vi "WholeImageROIFit.vi"(3 "Select directory with EYE files":path=path "E:/Focus Surgery/TTI LV Core") -> ()   [LabVIEW 2022 SP3]
uses:
  ViewData/-ReadEye/ScaleMethod.ctl
  <vilib>/Analysis/baseanly.llb/Mean (DBL).vi
  <vilib>/Utility/file.llb/Read Delimited Spreadsheet (DBL).vi
  <vilib>/Utility/file.llb/Write Delimited Spreadsheet (DBL).vi
  <vilib>/Analysis/NI_AALBase.lvlib
panel:
  out "Waveform Graph":cluster{"x-y":dbl, dbl, dbl[][]}(graph)
  out "spe vs depth":dbl[][](array[numeric])
  out "FileName":string
  in  "Color Scale":u16(ring) items=["Grey Scale", "Color Scale"]
  out "Sector as data array":dbl[][](graph)
  out "min value":dbl
  out "max value":dbl
  in  "ExitSendCmd":bool
  in  "Calculate TTIs":bool
  out "Current File":string
  out "Col scores":dbl[][](graph)
  out "Col midband":dbl[][](graph)
  out "NN Score":dbl[][](graph)
  in  "Tab Control":T1(tab)=enum."NNScore"
  in  "Type of Mean":u16(ring) items=["Mean from lines", "Mean just lines", "Poly Mean", "No mean", "Filter"]
  in  "Corrections":T2(ring)=enum."att correction"
  in  "type of cal file":u16(ring) items=["Normal Cal File", "Cross Cal File", "No cal file"]
  out "Cal File Att":string
  out "RF File Att":string
  out "Cal File Name":string
  in  "Fit band":T3 {"center freq" format="%.2f"; "stop freq" format="%.2f"; "start" format="%.2f"}
  in  "Use Info In Header?":bool=TRUE
  in  "Lines to Avg":i32=1
  in  "Pts between window":i32=8
  in  "Pts in window":i32=64
  in  "sound speed":dbl=1.5 format="%.2f"
  in  "Padded FFT size":u16(ring)=6 items=["next 2^n", "8", "16", "32", "64", "128", "256", "512"]
  in  "Att (db/ cm MHz)":dbl=0.5 format="%.2f"
  in  "Add Switch Noise?":bool
  in  "Log scaling?":T4=enum."Log Grey Scale"
  out "Fit array":T5
  in  "Define Att Start":bool
  out "window in mm":dbl
  in  "Axis scaling":bool
  out "dist between windows in mm":dbl
  in  "Sub-Band Filter":T6={"Fit band"={"low freq"=3.5, "high freq"=8.0, "center freq"=5.75}, "MB threshold"=0.0, "Sub-Band Filter?"=FALSE} {"MB threshold" format="%.2f"; "Fit band"."center freq" format="%.2f"; "Fit band"."high freq" format="%.2f"; "Fit band"."low freq" format="%.2f"}
  in  "Filter Prams":T7={"low cutoff"=5, "order"=81, "high cutoff"=35}
  in  "CQPrams":T8={"Data System params"={"sample freq (MHz)"=50.0, "focal length (mm)"=32.0, "aperature radius (mm)"=3.5, "pts in window"=64.0}, "Show CQ^2 image?"=FALSE, "Save?"=FALSE} {"Data System params"."pts in window" format="%.2f"; "Data System params"."aperature radius (mm)" format="%.2f"; "Data System params"."focal length (mm)" format="%.2f"; "Data System params"."sample freq (MHz)" format="%.2f"}
  out "CQ^2":ext[][](graph)
  out "radius (micron)":sgl[][](graph)
  in  "Range Params":T9={"mb max"=-20.0, "mb min"=-70.0, "slope max"=8.0, "slope min"=-8.0, "int max"=5.0, "int min"=-85.0} {"int min" format="%.2f"; "int max" format="%.2f"; "slope min" format="%.2f"; "slope max" format="%.2f"; "mb min" format="%.2f"; "mb max" format="%.2f"}
  in  "Final Sector Image Size":T10={"x"=346, "y"=240, "Trim image sides?"=FALSE, "start trim"=45, "end trim line"=256}
  in  "Simple BMP":bool
  in  "Raw Data Formats":T11(ring)
  in  "Save Raw Results?":bool
  out "inc x (mm)":dbl format="%.3f"
  out "inc y (mm)":dbl format="%.3f"
  out "Range Params in LUT":T9 {"int min" format="%.2f"; "int max" format="%.2f"; "slope min" format="%.2f"; "slope max" format="%.2f"; "mb min" format="%.2f"; "mb max" format="%.2f"}
  in  "Bypass Sector?":bool
  in  "PSA Value":dbl=8.7 format="%.2f"
  in  "Look Up Table":path=path "E:/Focus Surgery/TTI LV Core/99lktbl10-31.dat"
  in  "Create Score Image?":bool
  in  "thresholds":T12={"T1"=0.37, "T2"=0.38, "T3"=0.39, "T4"=0.4, "T5"=0.43} {"T5" scale=-0.1442227..0.5211197 scale format="%#_1g"; "T4" scale=-0.1442227..0.5211197 scale format="%#_1g"; "T3" scale=-0.1442227..0.5211197 scale format="%#_1g"; "T2" scale=-0.1442227..0.5211197 scale format="%#_1g"; "T1" scale=-0.1442227..0.6 scale format="%#_1g"}
  in  "Save Score Dat?":bool
  in  "Color Table":u32[](array[colorbox])=[0, 0, 65793, 131586, 197379, 263172, 328965, 394758, 460551, 526344, 592137, 657930, 723723, 789516, 855309, 921102, 986895, 1052688, 1118481, 1184274, 1250067, 1315860, 1381653, 1447446, 1513239, 1579032, 1644825, 1710618, 1776411, 1842204, 1907997, 1973790, 2039583, 2105376, 2171169, 2236962, 2302755, 2368548, 2434341, 2500134, 2565927, 2631720, 2697513, 2763306, 2829099, 2894892, 2960685, 3026478, 3092271, 3158064, 3223857, 3289650, 3355443, 3421236, 3487029, 3552822, 3618615, 3684408, 3750201, 3815994, 3881787, 3947580, 4013373, 4079166, 4144959, 4210752, 4276545, 4342338, 4408131, 4473924, 4539717, 4605510, 4671303, 4737096, 4802889, 4868682, 4934475, 5000268, 5066061, 5131854, 5197647, 5263440, 5329233, 5395026, 5460819, 5526612, 5592405, 5658198, 5723991, 5789784, 5855577, 5921370, 5987163, 6052956, 6118749, 6184542, 6250335, 6316128, 6381921, 6447714, 6513507, 6579300, 6645093, 6710886, 6776679, 6842472, 6908265, 6974058, 7039851, 7105644, 7171437, 7237230, 7303023, 7368816, 7434609, 7500402, 7566195, 7631988, 7697781, 7763574, 7829367, 7895160, 7960953, 8026746, 8092539, 8158332, 8224125, 8289918, 8355711, 8421504, 8487297, 8553090, 8618883, 8684676, 8750469, 8816262, 8882055, 8947848, 9013641, 9079434, 9145227, 9211020, 9276813, 9342606, 9408399, 9474192, 9539985, 9605778, 9671571, 9737364, 9803157, 9868950, 9934743, 10000536, 10066329, 10132122, 10197915, 10263708, 10329501, 10395294, 10461087, 10526880, 10592673, 10658466, 10724259, 10790052, 10855845, 10921638, 10987431, 11053224, 11119017, 11184810, 11250603, 11316396, 11382189, 11447982, 11513775, 11579568, 11645361, 11711154, 11776947, 11842740, 11908533, 11974326, 12040119, 12105912, 12171705, 12237498, 12303291, 12369084, 12434877, 12500670, 12566463, 12632256, 12698049, 12763842, 12829635, 12895428, 12961221, 13027014, 13092807, 13158600, 13224393, 13290186, 13355979, 13421772, 13487565, 13553358, 13619151, 13684944, 13750737, 13816530, 13882323, 13948116, 14013909, 14079702, 14145495, 14211288, 14277081, 14342874, 14408667, 14474460, 14540253, 14606046, 14671839, 14737632, 14803425, 14869218, 14935011, 15000804, 15066597, 15132390, 15198183, 15263976, 15329769, 15395562, 15461355, 15527148, 15592941, 15658734, 15724527, 15790320, 15856113, 15921906, 15987699, 16053492, 16119285, 16185078, 16250871, 16316664, 16382457, 6352640, 12058434, 16770066, 16758546, 16711731]
  in  "Data Set":i32
  in  "Rescale Thresh":bool
  in  "Save Cross Cal?":bool
  in  "Create Cross Cal?":bool
  out "Cross Cal":dbl[][](graph)
  in  "Avg #":i32=10
  out "avg":dbl[](array[numeric])
  in  "start avg":i32=270
  in  "AVG pts":i32=20
  in  "Save STFT AVG":bool
  in  "Ring":u16(ring) items=["Select Files in Listbox", "Choose list of files"]
  in  "File Names":i32[](listbox)
  out "raw data":i16[][](graph)
  out "midband fit":dbl[][](graph)
  out "intercept":dbl[][](graph)
  out "slope":dbl[][](graph)
  # "Z:\\_BIOMED_ARCHIVE\\Ex_Staff\\Andy_Kalisz_PC\\HITACHI\\HITACHI_2003-VMMC-CCal\\Andy_VMMC_2003-08-22_disk2\\Gel-cal\\EUP-V53W_End-Fire_Probe_SE13133935\\F3\\EYEfiles_-4dB"
  # "Z:\\_BIOMED_ARCHIVE\\DATA\\PROSTATE\\CALIBRATION AND X-CALIB\\NEW Data\\CrossCal Data - RRI Hitachi\\DG_2011-01-13"
  # "© 2000-2010 Riverside Research Institute"
  # "Parameters to select before hitting \"Calculate TTIs\"."
  # "Select to add back in switch noise from B&K Hawk machine."
  # "Spectrum Fit Parameters"
  # "Values used to make image."
  # "Optional suband filter which is really never used and may not function properly in current version."
  # "Can be selected after calculating TTIs"
  # "CQPrams files are saved as spreadsheet files. Radius file is in microns and cq^2 file is in dB."
  # "Pixel spacing of sector image.\n(Need to be same for 1:1 aspect ration.)"
  # "Save raw data and MB side by side"
  # "Score images need to be created with all corrections applied data. This means a cross cal file with attenutation corrections for Hawk and Hitachi, and data base corrections for B&K 3535.\n\nFinal image size settings are in Image Prams tab. Data saves as a BMP file in sector format.\n\nCreate Score Image? will color code images and Save Score Dat? will save images as BMPs."
  # "If making Cross Cal file, select No cal file option and att correction."
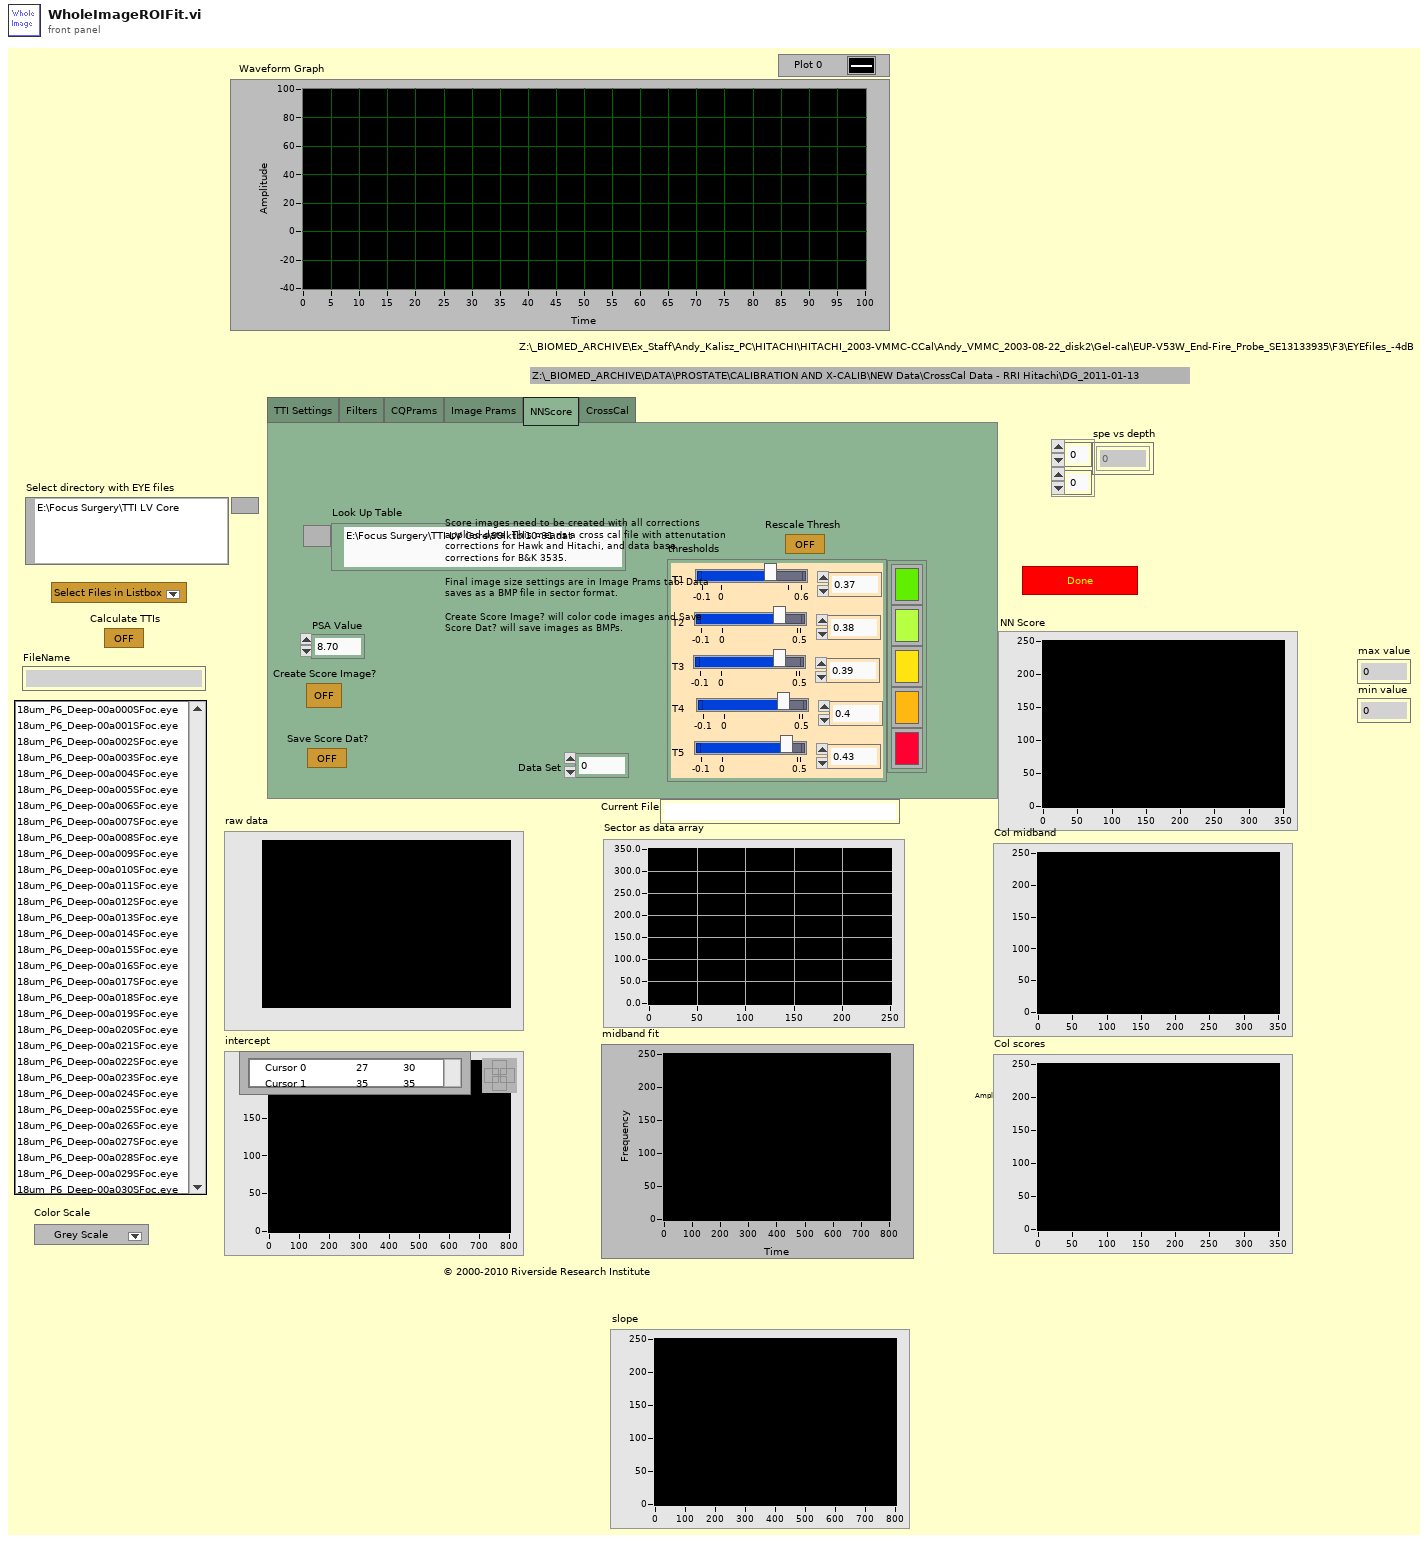
[diagram p1: front panel]
types:
  T1 = enum32{"TTI Settings", "Filters", "CQPrams", "Image Prams", "NNScore", "CrossCal"}
  T2 = enum16{"no att correction", "att correction", "B&K 3535, TGC & att corr"}
  T3 = cluster{"start":dbl, "stop freq":dbl, "center freq":dbl}
  T4 = typedef "ScaleMethod.ctl" = enum16{"Linear Abs Grey", "Log Grey Scale", "Linear Color Scale", "dB Scale", "Verasonics Doppler"}
  T5 = cluster{"x length":i32, "y length":i32, "ROIs in x":i32, "ROIs in y":i32}
  T6 = cluster{"Fit band":cluster{"low freq":dbl, "high freq":dbl, "center freq":dbl}, "MB threshold":dbl, "Sub-Band Filter?":bool}
  T7 = cluster{"low cutoff":i32, "order":i32, "high cutoff":i32}
  T8 = cluster{"Data System params":cluster{"sample freq (MHz)":dbl, "focal length (mm)":sgl, "aperature radius (mm)":sgl, "pts in window":dbl}, "Show CQ^2 image?":bool, "Save?":bool}
  T9 = cluster{"mb max":dbl, "mb min":dbl, "slope max":dbl, "slope min":dbl, "int max":dbl, "int min":dbl}
  T10 = cluster{"x":i32, "y":i32, "Trim image sides?":bool, "start trim":i32, "end trim line":i32}
  T11 = enum16{"spreadsheet", "8 bit byte file", "sector byte file", "8 bit BMP file", "sector 8 bit BMP file"}
  T12 = cluster{"T1":dbl, "T2":dbl, "T3":dbl, "T4":dbl, "T5":dbl}
  T13 = typedef "Header.ctl" = cluster{"header info":cluster{"Header":string, "Head length":i16}, "A/D info":cluster{"# rf points per line":u16, "# lines per scan":u16, "sample rate MHz":u16, "# A/D bits":i16, "# bytes per A/D":u16, "TGC Flag":u16, "A/D Type":string}, "Tranducer Info":cluster{"bandwidth":sgl, "center freq":sgl, "start freq":sgl, "ID":i32}, "Scan Info":cluster{"delay":sgl, "pivot distance":sgl, "sector scan angle":sgl, "operator":string, "Scan Mode":string, "location":string}, "Time/Date Info":cluster{"date":string, "time":string}, "RF Info":cluster{"RF file name":string, "RF file att":string, "RF cal file name":string, "RF cal file att":string}, "Patient Info":cluster{"ID":string, "extended ID":string, "age":u16, "sex":string, "previously\nscanned":string, "PSA":sgl, "LOS":u8, "Ethnicty 2":u8, "Race":u8}, "Tissue Type":cluster{"organ":i16, "disease type":i16, "disease location":i16, "IQ_pts":u16, "RcvBuffer":u8, "RcvFrame":u16, "IQBuff":u8, "IQFrame":u16, "IQPage":u8}, "Votage scaling":cluster{"Digitizer (dB)":sgl, "Gain (dB)":sgl, "Atten (dB)":sgl}, "Comment":string, "Misc Info":cluster{"avg num":u16, "c speed":i16, "Div By or SF zones":i16, "XMIT CHS":u8, "RCV CHS":u8, "Xmit angle":sgl}, "Therapy Parameters":cluster{"Theraputic Freq (MHz)":sgl, "Time on (s)":sgl, "Therapy amplitude (mV)":sgl, "Lines Before":u16, "Lines After":u16}, "Scan Settings":cluster{"Energy (uJ or V)":u8, "Damp (Ohm) or Fc":u8, "HP Filt (KHz)":u8, "LP Filt (MHz)":u8, "Gain (db)":u8, "prf (kHz)":sgl, "Distance between\nscan lines (um)":u16, "Distance between\nscan planes (um)":u16, "Scan line gap (um)":sgl, "Scan plane gap (um)":sgl}, "Compression Parameters":cluster{"F1 (MHz)":sgl, "F2 (MHz)":sgl, "% taper":sgl, "duration":sgl}, "Patient Info Xtra":cluster{"First Name":string, "Last Name":string, "Notes":string}, "ROI Box":u16[]}
  T14 = cluster{"delay":sgl, "pivot distance":sgl, "sector scan angle":sgl, "operator":string, "Scan Mode":string, "location":string}
  T15 = cluster{"X right":dbl, "X left":dbl, "Y low":dbl, "Y high":dbl}
  T16 = cluster{"RF file name":string, "RF File Att":string, "Cal File Name":string, "Cal File Att":string}
  T17 = cluster{"RF file name":string, "RF file att":string, "RF cal file name":string, "RF cal file att":string}
  T18 = cluster{"start freq":sgl, sgl, "center freq":sgl}
  T19 = cluster{"bandwidth":sgl, "center freq":sgl, "start freq":sgl, "ID":i32}
  T20 = cluster{"Pts in window":i32, "Lines to Avg":i32, dbl, "# lines per scan":u16}
  T21 = cluster{"slope (m)":dbl[][], "intercept (b)":dbl[][], "midband fit":dbl[][], "pts in fit":dbl}
  T22 = cluster{"slope (m)":dbl, "m stand dev":dbl, "intercept (b)":dbl, "b stand dev":dbl, "MSE":dbl, "midband fit":dbl, "pts in fit":dbl}
  T23 = typedef "imagedata.ctl" = cluster{"image type":i32, "image depth":i32, "image":u8[], "mask":u8[], "colors":u32[], "Rectangle":cluster{"left":i16, "top":i16, "right":i16, "bottom":i16}}
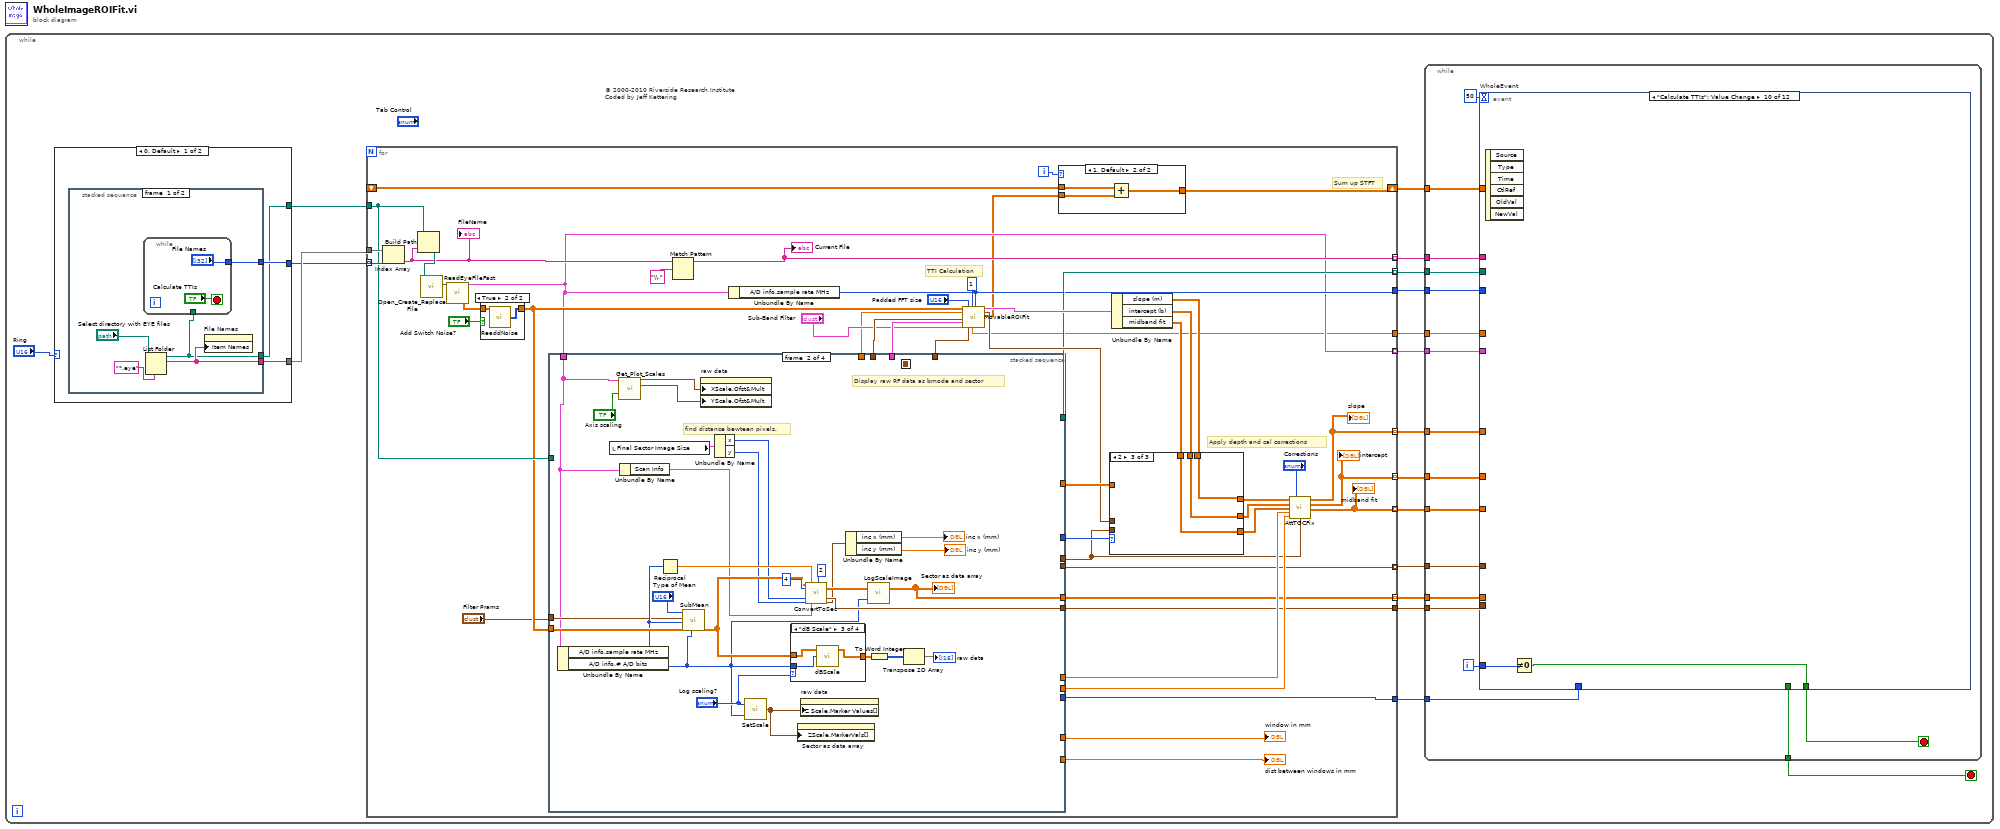
[diagram p0: block diagram]
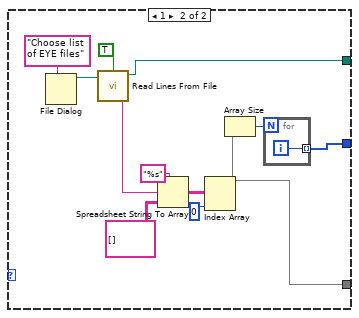
[diagram p3: hidden frame]
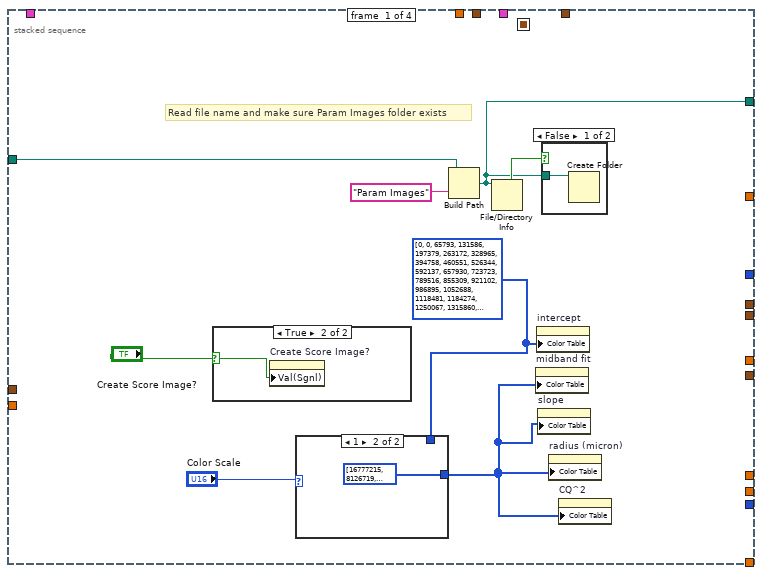
[diagram p5: hidden frame]
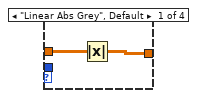
[diagram p9: hidden frame]
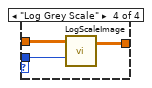
[diagram p11: hidden frame]
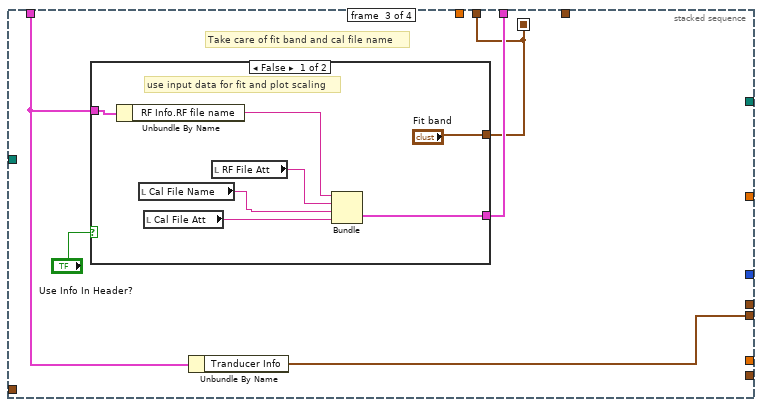
[diagram p12: hidden frame]
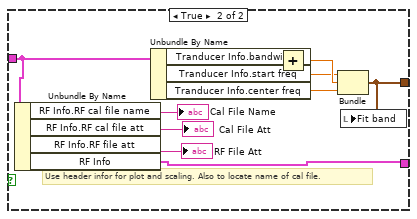
[diagram p13: hidden frame]
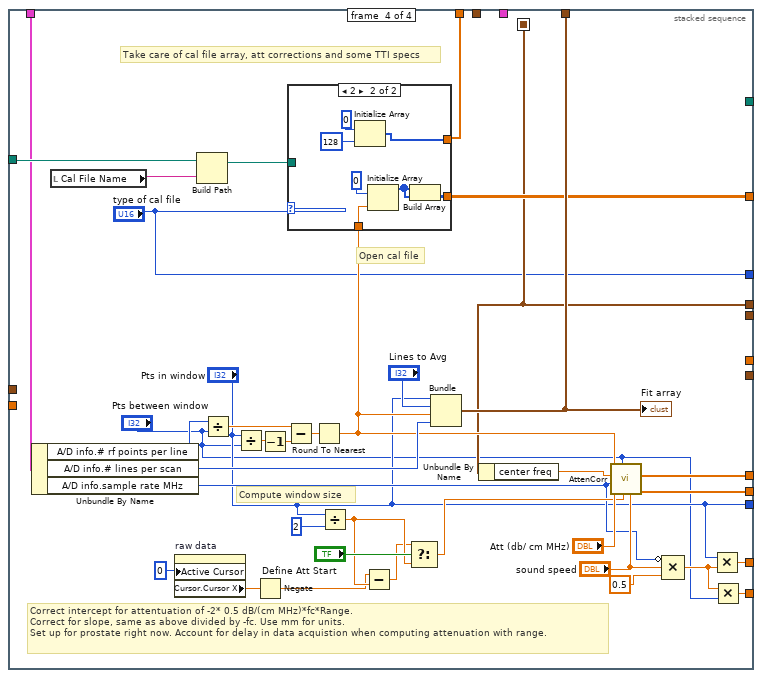
[diagram p14: hidden frame]
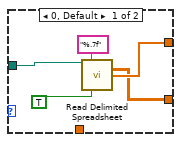
[diagram p15: hidden frame]
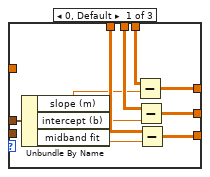
[diagram p17: hidden frame]
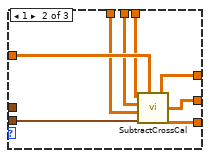
[diagram p18: hidden frame]
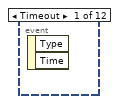
[diagram p19: hidden frame]
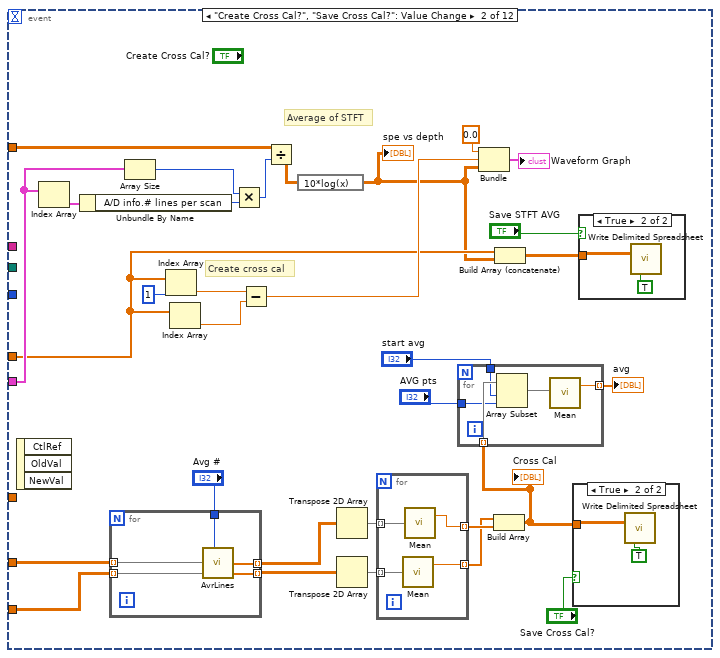
[diagram p20: hidden frame]
diagram:
  n1 = while {
    stop <- w5 stop-if-true
    # "© 2000-2010 Riverside Research Institute\nCoded by Jeff Kettering"
    n2 = case shown="0, Default" "Ring" {
      tunnel: [w21 w31] -> w18
      tunnel: [w20 w30] -> w17
      tunnel: [w19 w29] -> w4
      frame 0, Default {
        n3 = stacked-sequence {
          tunnel: [w23 _] -> w21
          tunnel: [w24 _] -> w20
          tunnel: [w22 _] -> w19
          frame #0 {
            n4 = List Folder(path="Select directory with EYE files", pattern="*.eye") -> (path out=w22:path, filenames=w23:string[])  [unwired: 1 in, 3 out]
            n5 = while {
              tunnel: ["File Names"] -> w24
              tunnel: w22 -> [_]
              stop <- "Calculate TTIs" stop-if-true
            }
            n6 = property on="File Names" class="LstBox (strict)"("Item Names"=w23) -> ()  [unwired: 2 in, 2 out]
          }
          frame #1 {
          }
        }
      }
      frame 1 {
        n7 = File Dialog(7:"Choose list of EYE files" ("prompt")) -> (3:w38:path)  [unwired: 1 in, 8 out]
        n8 = call <vilib>:"Read Lines From File.vi"("convert eol? (no:F)"=TRUE, "file path (dialog if empty)"=w38) -> ("new file path (Not A Path if cancelled)"=w29:path, "line string"=w33:string)  [unwired: 1 in, 5 out]
        n9 = Spreadsheet String To Array(format string="%s", spreadsheet string=w33, array type (2D Dbl)=string[][] [] ("Array Constant")) -> (array=w37:string[][])  [unwired: 1 in]
        n10 = Index Array(array=w37, index (col)=0) -> (element=w31:string[])  [unwired: 1 in]
        n11 = Array Size(array=w31) -> (size(s)=w32:i32)
        n12 = for {
          N: w32 -> [_]
          tunnel: [w41] -> w30 mode=indexing
          i -> [w41]
        }
      }
    }
    n13 = for {
      tunnel: w18 -> [w88]
      tunnel: w4 -> [w66]
      tunnel: w17 -> [w86] mode=indexing
      tunnel: [w60] -> w16 mode=indexing
      tunnel: [w67] -> w15 mode=indexing
      tunnel: [w56] -> w14 mode=indexing
      tunnel: [w54] -> w13 mode=indexing
      tunnel: [w68] -> w12 mode=indexing
      tunnel: [w55] -> w11 mode=indexing
      tunnel: [w51] -> w10 mode=indexing
      tunnel: [w65] -> w9
      tunnel: [w59] -> w8 mode=indexing
      tunnel: [w52] -> w7
      tunnel: [w57] -> w6
      shift-right: [w42] -> w2
      shift-left: _ -> [w47]
      tunnel: [w49] -> w1
      i -> [w46]
      # "Sum up STFT"
      # "Apply depth and cal corrections"
      # "TTI Calculation"
      n14 = Index Array(array=w88, index=w86) -> (element=w61:string)
      "FileName" <- w61
      n15 = Build Path(base path=w66, name or relative path=w61) -> (appended path=w87:path)
      n16 = call <vilib>:"Open_Create_Replace File.vi"("file path"=w87) -> ("new file path"=w72:path)  [unwired: 5 in, 5 out]
      n17 = call "ReadEyeFileFast.vi"("new file path"=w72) -> ("2-D data array"=w58:sgl[][], "Header In"=w51:T13)  [unwired: 13 in, 4 out]
      n18 = case shown="True" "Add Switch Noise?" {
        tunnel: [w216 w218] -> w63
        tunnel: w58 -> [w216 w217]
        frame False {
        }
        frame True {
          n19 = call "ReaddNoise.vi"("Data in"=w217) -> ("Data out"=w218:i16[][])
        }
      }
      n20 = stacked-sequence {
        seq-local: [_ _ w145 _] -> [_ _ _ w184]
        tunnel: [_ _ _ w203] -> w43
        tunnel: [_ _ w148 _] -> w89
        tunnel: w66 -> [w99 _ _ w193]
        tunnel: [_ _ _ w192] -> w79
        tunnel: [_ _ _ w191] -> w78
        tunnel: [_ _ _ w190] -> w50
        tunnel: [_ _ _ "type of cal file"] -> w76
        tunnel: [_ _ _ w187] -> w75
        tunnel: [_ _ w145 _] -> w70
        tunnel: [_ _ _ w184] -> w69
        tunnel: [_ _ w146 _] -> w68
        tunnel: [w101 _ _ _] -> w67
        tunnel: [_ w125 _ _] -> w65
        tunnel: w63 -> [_ w124 _ _]
        tunnel: [_ w123 _ _] -> w59
        tunnel: [_ _ _ "Pts in window"] -> w57
        tunnel: "Filter Prams" -> [_ w120 _ _]
        tunnel: w51 -> [_ w112 w147 w175]
        tunnel: [_ _ _ w170] -> w45
        tunnel: [_ _ _ w167] -> w44
        frame #0 {
          w97 = u32[] [0, 0, 65793, 131586, 197379, 263172, 328965, 394758, 460551, 526344, 592137, 657930, 723723, 789516, 855309, 921102, 986895, 1052688, 1118481, 1184274, 1250067, 1315860, 1381653, 1447446, 1513239, 1579032, 1644825, 1710618, 1776411, 1842204, 1907997, 1973790, 2039583, 2105376, 2171169, 2236962, 2302755, 2368548, 2434341, 2500134, 2565927, 2631720, 2697513, 2763306, 2829099, 2894892, 2960685, 3026478, 3092271, 3158064, 3223857, 3289650, 3355443, 3421236, 3487029, 3552822, 3618615, 3684408, 3750201, 3815994, 3881787, 3947580, 4013373, 4079166, 4144959, 4210752, 4276545, 4342338, 4408131, 4473924, 4539717, 4605510, 4671303, 4737096, 4802889, 4868682, 4934475, 5000268, 5066061, 5131854, 5197647, 5263440, 5329233, 5395026, 5460819, 5526612, 5592405, 5658198, 5723991, 5789784, 5855577, 5921370, 5987163, 6052956, 6118749, 6184542, 6250335, 6316128, 6381921, 6447714, 6513507, 6579300, 6645093, 6710886, 6776679, 6842472, 6908265, 6974058, 7039851, 7105644, 7171437, 7237230, 7303023, 7368816, 7434609, 7500402, 7566195, 7631988, 7697781, 7763574, 7829367, 7895160, 7960953, 8026746, 8092539, 8158332, 8224125, 8289918, 8355711, 8421504, 8487297, 8553090, 8618883, 8684676, 8750469, 8816262, 8882055, 8947848, 9013641, 9079434, 9145227, 9211020, 9276813, 9342606, 9408399, 9474192, 9539985, 9605778, 9671571, 9737364, 9803157, 9868950, 9934743, 10000536, 10066329, 10132122, 10197915, 10263708, 10329501, 10395294, 10461087, 10526880, 10592673, 10658466, 10724259, 10790052, 10855845, 10921638, 10987431, 11053224, 11119017, 11184810, 11250603, 11316396, 11382189, 11447982, 11513775, 11579568, 11645361, 11711154, 11776947, 11842740, 11908533, 11974326, 12040119, 12105912, 12171705, 12237498, 12303291, 12369084, 12434877, 12500670, 12566463, 12632256, 12698049, 12763842, 12829635, 12895428, 12961221, 13027014, 13092807, 13158600, 13224393, 13290186, 13355979, 13421772, 13487565, 13553358, 13619151, 13684944, 13750737, 13816530, 13882323, 13948116, 14013909, 14079702, 14145495, 14211288, 14277081, 14342874, 14408667, 14474460, 14540253, 14606046, 14671839, 14737632, 14803425, 14869218, 14935011, 15000804, 15066597, 15132390, 15198183, 15263976, 15329769, 15395562, 15461355, 15527148, 15592941, 15658734, 15724527, 15790320, 15856113, 15921906, 15987699, 16053492, 16119285, 16185078, 16250871, 16316664, 16382457, 16448250, 16514043, 16579836, 16645629, 16711680] ("Color Table")
          # "Read file name and make sure Param Images folder exists"
          n21 = case shown="True" "Create Score Image?" {
            selector: "Create Score Image?" -> [_ w106]
            frame False {
            }
            frame True {
              n22 = property on="Create Score Image?" class="Bool (strict)"("Val(Sgnl)"=w106) -> ()  [unwired: 2 in, 2 out]
            }
          }
          n23 = case shown="1" "Color Scale" {
            tunnel: [w104 u32[] [16777215, 8126719, 7864574, 7536895, 7274750, 6947071, 6684926, 6357247, 6095102, 5767423, 5505278, 5177599, 4915454, 4587775, 4325630, 3997951, 3735806, 3408127, 3145982, 2818303, 2556158, 2228479, 1966334, 1638655, 1376510, 1048831, 786686, 459007, 196862, 767, 1790, 3071, 4094, 5375, 6398, 7679, 8702, 9983, 11006, 12287, 13310, 14591, 15614, 16895, 17918, 19199, 20222, 21503, 22526, 23807, 24830, 26111, 27134, 28415, 29438, 30719, 31486, 33023, 33790, 35327, 36094, 37631, 38398, 39935, 40702, 42239, 43006, 44543, 45310, 46847, 47614, 49151, 49918, 51455, 52222, 53759, 54526, 56063, 56830, 58367, 59134, 60671, 61694, 62975, 63998, 65279, 65274, 65527, 65265, 65518, 65256, 65509, 65247, 65500, 65238, 65491, 65229, 65482, 65220, 65473, 65211, 65464, 65202, 65455, 65193, 65446, 65184, 65437, 65175, 65428, 65166, 65419, 65157, 65410, 65149, 65401, 65140, 65392, 65131, 65383, 65122, 65374, 65113, 65365, 65104, 65356, 65095, 65347, 65086, 65338, 65077, 65329, 65068, 65320, 65059, 65311, 65050, 65302, 65041, 65293, 65032, 65284, 130560, 392960, 720384, 982784, 1310208, 1572608, 1900032, 2162432, 2489856, 2752256, 3079680, 3342080, 3669504, 3931904, 4259328, 4521728, 4849152, 5111552, 5438976, 5701376, 6028800, 6291200, 6618624, 6881024, 7208448, 7470848, 7798272, 8126208, 8322560, 8716032, 8912384, 9305856, 9502208, 9895680, 10092032, 10485504, 10681856, 11075328, 11271680, 11665152, 11861504, 12254976, 12451328, 12844800, 13041152, 13434624, 13630976, 14024448, 14220800, 14614272, 14810624, 15204096, 15400448, 15793920, 15990272, 16383744, 16580096, 16776192, 16709376, 16773888, 16707072, 16771584, 16704768, 16769280, 16702464, 16766976, 16700160, 16764672, 16697856, 16762368, 16695552, 16760064, 16693248, 16757760, 16690944, 16755456, 16688640, 16753152, 16686336, 16750848, 16684032, 16748544, 16681728, 16746240, 16679680, 16743936, 16677376, 16741632, 16675072, 16739328, 16672768, 16737024, 16670464, 16734720, 16668160, 16732416, 16665856, 16730112, 16663552, 16727808, 16661248, 16725504, 16658944, 16723200, 16656640, 16720896, 16654336, 16718592, 16652032, 16716288, 16649728, 16713984, 16712960, 0] ("256 log up 2")] -> w96
            tunnel: w97 -> [w104 _]
            frame 0, Default {
            }
            frame 1 {
            }
          }
          n24 = Build Path(base path=w99, name or relative path="Param Images") -> (appended path=w101:path)
          n25 = File/Directory Info(path=w101) -> (directory=w103:bool)  [unwired: 1 in, 6 out]
          n26 = property on="midband fit" class="IntGraph (strict)"("Color Table"=w96) -> ()  [unwired: 2 in, 2 out]
          n27 = property on="intercept" class="IntGraph (strict)"("Color Table"=w97) -> ()  [unwired: 2 in, 2 out]
          n28 = property on="slope" class="IntGraph (strict)"("Color Table"=w96) -> ()  [unwired: 2 in, 2 out]
          n29 = case shown="False" w103 {
            tunnel: w101 -> [w107 _]
            frame False {
              n30 = Create Folder(path (use dialog)=w107) -> ()  [unwired: 1 in, 4 out]
            }
            frame True {
            }
          }
          n31 = property on="radius (micron)" class="IntGraph (strict)"("Color Table"=w96) -> ()  [unwired: 2 in, 2 out]
          n32 = property on="CQ^2" class="IntGraph (strict)"("Color Table"=w96) -> ()  [unwired: 2 in, 2 out]
        }
        frame #1 {
          # "find distance bewteen pixels."
          # "Display raw RF data as bmode and sector"
          n33 = Unbundle By Name(w112) -> ("A/D info.sample rate MHz"=w121:u16, "A/D info.# A/D bits"=w108:i16)
          n34 = local read "Final Sector Image Size"() -> (w126:T10)
          n35 = call "Get_Plot_Scales.vi"("Header In"=w112, "Axis scaling"="Axis scaling") -> ("Depth Scale"=w111:cluster{"start depth":dbl, "depth interval":dbl}, "Width Scale"=w110:cluster{"Start":dbl, "width Interval":dbl})  [unwired: 12 in]
          n36 = Unbundle By Name(w112) -> ("Scan Info"=w118:T14)
          n37 = Reciprocal(x=w121) -> (1/x=w133:dbl)
          n38 = call "SubMean.vi"("Bit Depth"=w108, "Scan Data In"=w124, "Samp Rate (MHz)"=w121, "Filter Prams"=w120, "Type of Mean"="Type of Mean") -> ("Array"=w127:dbl[][])  [unwired: 1 in, 2 out]
          n39 = property on="raw data" class="IntGraph (strict)"("XScale.Ofst&Mult"=w111, "YScale.Ofst&Mult"=w110) -> ()  [unwired: 2 in, 2 out]
          n40 = Unbundle By Name(w126) -> ("x"=w117:i32, "y"=w116:i32)
          n41 = call "SetScale.vi"("# A/D bits"=w108, "Display mode"="Log scaling?") -> ("Array"=w131:cluster{dbl, u32}[])
          n42 = case shown="\"dB Scale\"" "Log scaling?" {
            tunnel: [w137 w138 w140 w144] -> w130
            tunnel: w127 -> [w136 w138 w141 w143]
            tunnel: w108 -> [_ _ w139 w142]
            frame "Linear Abs Grey", Default {
              n43 = Absolute Value(x=w136) -> (abs(x)=w137:dbl[][])
            }
            frame "Linear Color Scale" {
            }
            frame "dB Scale" {
              n44 = call "dBScale.vi"("Bit Depth"=w139, "Data In"=w141) -> ("Data Out"=w140:dbl[][])  [unwired: 3 in]
            }
            frame "Log Grey Scale" {
              n45 = call "LogScaleImage.vi"("A/D bits"=w142, "input array"=w143) -> ("log scale image"=w144:dbl[][])  [unwired: 1 out]
            }
          }
          n46 = property on="Sector as data array" class="IntGraph (strict)"("ZScale.MarkerVals[]"=w131) -> ()  [unwired: 2 in, 2 out]
          n47 = property on="raw data" class="IntGraph (strict)"("Z Scale.Marker Values[]"=w131) -> ()  [unwired: 2 in, 2 out]
          n48 = call "ConvertToSec.vi"("raw image data in"=w127, "reduce pts by factor of"=4, "pixels in x"=w117, "pixels in y"=w116, "Time between rf pts\nmicros"=w133, "Scan Info"=w118, "Smooth factor"=2) -> ("raw sector out"=w132:dbl[][], "Axis scaling Params"=w125:T15, "scales"=w115:cluster{"inc x (mm)":dbl, "inc y (mm)":dbl})  [unwired: 4 in, 6 out]
          n49 = Unbundle By Name(w115) -> ("inc x (mm)"=→"inc x (mm)":dbl, "inc y (mm)"=→"inc y (mm)":dbl)
          n50 = call "LogScaleImage.vi"("A/D bits"=w108, "input array"=w132) -> ("log scale image"=w123:dbl[][])  [unwired: 1 out]
          "Sector as data array" <- w123
          n51 = To Word Integer(number=w130) -> (16bit integer=w129:i16[][])
          n52 = Transpose 2D Array(2D array=w129) -> (transposed array=→"raw data":i16[][])
        }
        frame #2 {
          # "Take care of fit band and cal file name"
          n53 = case shown="False" "Use Info In Header?" {
            tunnel: w147 -> [w150 w158]
            tunnel: ["Fit band" w162] -> w145
            tunnel: [w155 w157] -> w148
            frame False {
              # "use input data for fit and plot scaling"
              n54 = Unbundle By Name(w150) -> ("RF Info.RF file name"=w156:string)
              n55 = local read "Cal File Name"() -> (w151:string)
              n56 = local read "Cal File Att"() -> (w152:string)
              n57 = local read "RF File Att"() -> (w153:string)
              n58 = Bundle("RF file name"=w156, "RF File Att"=w153, "Cal File Name"=w151, "Cal File Att"=w152) -> (w155:T16)  [unwired: 1 out]
            }
            frame True {
              # "Use header infor for plot and scaling. Also to locate name of cal file."
              n59 = Unbundle By Name(w158) -> ("RF Info.RF cal file name"=→"Cal File Name":string, "RF Info.RF cal file att"=→"Cal File Att":string, "RF Info.RF file att"=→"RF File Att":string, "RF Info"=w157:T17)
              n60 = Unbundle By Name(w158) -> ("Tranducer Info.bandwidth"=w166:sgl, "Tranducer Info.start freq"=w163:sgl, "Tranducer Info.center freq"=w165:sgl)
              n61 = Add(x=w166, y=w163) -> (x+y=w164:sgl)
              n62 = Bundle("start freq"=w163, w164, "center freq"=w165) -> (w162:T18)  [unwired: 1 out]
              n63 = local write "Fit band"(w162) -> ()
            }
          }
          n64 = Unbundle By Name(w147) -> ("Tranducer Info"=w146:T19)
        }
        frame #3 {
          # "Correct intercept for attentuation of -2* 0.5 dB/(cm MHz)*fc*Range.\nCorrect for slope, same as above divided by -fc. Use mm for units. \nSet up for prostate right now. Account for delay in data acquistion when computing attenuation with range."
          # "Take care of cal file array, att corrections and some TTI specs"
          # "Compute window size"
          # "Open cal file"
          n65 = Unbundle By Name(w175) -> ("A/D info.# rf points per line"=w199:u16, "A/D info.# lines per scan"=w189:u16, "A/D info.sample rate MHz"=w172:u16)
          n66 = local read "Cal File Name"() -> (w186:string)
          n67 = property on="raw data" class="IntGraph (strict)"("Active Cursor"=u32 0) -> ("Cursor.Cursor X"=w181:dbl)  [unwired: 2 in, 2 out]
          n68 = Build Path(base path=w193, name or relative path=w186) -> (appended path=w202:path)
          n69 = Divide(x=w199, y="Pts between window") -> (x/y=w201:dbl)
          n70 = Divide(x="Pts in window", y="Pts between window") -> (x/y=w196:dbl)
          n71 = Negate(x=w181) -> (-x=w177:dbl)
          n72 = Decrement(x=w196) -> (x-1=w195:dbl)
          n73 = Subtract(x=w201, y=w195) -> (x-y=w200:dbl)
          n74 = Round To Nearest(number=w200) -> (nearest integer value=w188:dbl)
          n75 = case shown="2" "type of cal file" {
            tunnel: w202 -> [w208 _]
            tunnel: [w205 w213] -> w203
            tunnel: [w204 w209] -> w187
            tunnel: w188 -> [_ w212]
            frame 0, Default {
              n76 = call-poly <vilib>:"Read Delimited Spreadsheet.vi"("file path (dialog if empty)"=w208, "format (%.3f)"="%.7f", "transpose? (F)"=TRUE ("transpose (no:F)")) -> ("all rows"=w204:dbl[][], "first row"=w205:dbl[])  [unwired: 7 in, 4 out]
            }
            frame 2 {
              n77 = Initialize Array(0, 128) -> (w213:i32[])
              n78 = Initialize Array(0, w212) -> (w210:i32[])
              n79 = Build Array(w210, w210) -> (w209:i32[][])
            }
          }
          n80 = Divide(x="Pts in window", y=2) -> (x/y=w178:dbl)
          n81 = Subtract(x=w177, y=w178) -> (x-y=w176:dbl)
          n82 = Select(t=w176, s="Define Att Start", f=w178) -> (s? t:f=w182:dbl)
          n83 = Bundle("Pts in window"="Pts in window", "Lines to Avg"="Lines to Avg", w188, "# lines per scan"=w189) -> (w190:T20)  [unwired: 1 out]
          "Fit array" <- w190
          n84 = Unbundle By Name(w184) -> ("center freq"=w198:dbl)
          n85 = call "AttenCorr.vi"("sound speed"="sound speed", "Offset"=w182, "Step size"="Pts between window", "Attenuation (db/ cm MHz)"="Att (db/ cm MHz)", "Sampling Freq (MHz)"=w172, "Center Freq"=w198, "ROIs in x"=w188) -> ("slope correction"=w191:dbl[], "midband correction"=w192:dbl[])  [unwired: 2 out]
          n86 = Compound Arithmetic op=MULTIPLY(invert w172, "sound speed", 0.5 ("value")) -> (w169:dbl)
          n87 = Multiply(x="Pts in window", y=w169) -> (x*y=w170:dbl)
          n88 = Multiply(x=w169, y="Pts between window") -> (x*y=w167:dbl)
        }
      }
      "window in mm" <- w45
      "dist between windows in mm" <- w44
      n89 = Match Pattern(string=w61, regular expression="\\." ("search char (-)")) -> (before substring=w60:string)  [unwired: 4 out]
      "Current File" <- w60
      n90 = Unbundle By Name(w51) -> ("A/D info.sample rate MHz"=w52:u16)
      n91 = call "MovableROIFit.vi"("input array"=w63, "calibration data"=w43, "Fit band"=w70, "RF Info"=w89, "Sub-Band Filter"="Sub-Band Filter", "FFT size for"="Padded FFT size", "Fit array"=w50, "Proc Method"=1, "freq (MHz)"=w52) -> ("Freq Values"=w49:dbl[], "Raw Fit Data"=w90:T21, "Cal params"=w71:T22, "STFT Sum"=w48:dbl[][])  [unwired: 4 in, 3 out]
      n92 = case shown="1, Default" w46 {
        tunnel: w48 -> [w92 w93]
        tunnel: w47 -> [_ w95]
        tunnel: [w92 w94] -> w42
        frame 0 {
        }
        frame 1, Default {
          n93 = Add(x=w95, y=w93) -> (x+y=w94:dbl[][])
        }
      }
      n94 = Unbundle By Name(w90) -> ("slope (m)"=w83:dbl[][], "intercept (b)"=w84:dbl[][], "midband fit"=w85:dbl[][])
      n95 = case shown="2" w76 {
        tunnel: w71 -> [w228 _ _]
        tunnel: w85 -> [w227 w231 w238]
        tunnel: [w226 w235 w238] -> w80
        tunnel: w84 -> [w225 w230 w239]
        tunnel: [w224 w234 w239] -> w81
        tunnel: w83 -> [w223 w229 w237]
        tunnel: [w222 w233 w237] -> w82
        tunnel: w69 -> [_ w236 _]
        tunnel: w75 -> [_ w232 _]
        frame 0, Default {
          n96 = Unbundle By Name(w228) -> ("slope (m)"=w221:dbl, "intercept (b)"=w220:dbl, "midband fit"=w219:dbl)
          n97 = Subtract(x=w223, y=w221) -> (x-y=w222:dbl[][])
          n98 = Subtract(x=w225, y=w220) -> (x-y=w224:dbl[][])
          n99 = Subtract(x=w227, y=w219) -> (x-y=w226:dbl[][])
        }
        frame 1 {
          n100 = call "SubtractCrossCal.vi"("slope (m)"=w229, "intercept (b) out"=w230, "midband fit in"=w231, "Fit band"=w236, "Cross Cal"=w232) -> ("slope out"=w233:dbl[][], "intercept out"=w234:dbl[][], "midband fitout"=w235:dbl[][])
        }
        frame 2 {
        }
      }
      n101 = call "AttTGCFix.vi"("slope (m)"=w82, "Corrections"="Corrections", "intercept (b) out"=w81, "midband fit in"=w80, "midband correction"=w79, "slope correction"=w78, "Fit band"=w69) -> ("slope"=w56:dbl[][], "intercept"=w55:dbl[][], "midband fit"=w54:dbl[][])  [unwired: 6 out]
      "intercept" <- w55
      "slope" <- w56
      "midband fit" <- w54
    }
    n102 = while {
      tunnel: w16 -> [w256]
      tunnel: w15 -> [w255]
      tunnel: w14 -> [w254]
      tunnel: w13 -> [w253]
      tunnel: w12 -> [w252]
      tunnel: w11 -> [w251]
      tunnel: w10 -> [w250]
      tunnel: w9 -> [w248]
      tunnel: w8 -> [w247]
      tunnel: w7 -> [w246]
      tunnel: w6 -> [w245]
      tunnel: [w243] -> w5
      tunnel: w2 -> [w242]
      tunnel: w1 -> [w241]
      i -> [w240]
      stop <- w244 stop-if-true
      n103 = event "WholeEvent" shown="[9] \"Calculate TTIs\": Value Change" {
        selector: _ -> [_ _ _ _ _ _ _ _ _ _ _ _]
        dyn-events: _ -> [_ _ _ _ _ _ _ _ _ _ _ _]
        timeout: 50 -> [_ _ _ _ _ _ _ _ _ _ _ _]
        tunnel: w256 -> [_ _ w314 w328 w341 w364 w384 _ _ _ _ _]
        tunnel: w255 -> [_ _ w312 w332 w342 _ w385 _ _ _ _ _]
        tunnel: w254 -> [_ _ w310 w331 _ _ _ _ _ _ _ _]
        tunnel: w253 -> [_ w281 w308 w330 _ w366 w381 _ _ _ _ _]
        tunnel: w252 -> [_ _ _ w329 _ _ _ _ _ _ _ _]
        tunnel: w251 -> [_ w282 w309 _ _ w367 w382 _ _ _ _ _]
        tunnel: w250 -> [_ w271 w311 _ _ w365 w383 _ _ _ _ _]
        tunnel: [_ _ _ _ _ _ _ _ TRUE w404 w406 _] -> w244
        tunnel: w248 -> [_ _ _ _ _ _ _ _ _ _ _ w407]
        tunnel: w247 -> [_ _ _ _ _ w358 _ _ _ _ _ _]
        tunnel: w246 -> [_ _ _ w326 _ _ _ _ _ _ _ _]
        tunnel: w245 -> [_ _ _ w325 _ _ _ _ _ _ _ _]
        tunnel: [_ _ _ _ _ _ _ _ _ _ w406 _] -> w243
        tunnel: w242 -> [_ w273 _ _ _ _ _ _ _ _ _ _]
        tunnel: w241 -> [_ w260 _ _ _ _ _ _ _ _ _ _]
        tunnel: w240 -> [_ _ _ _ _ _ _ _ _ w405 _ _]
        event Timeout {
          n104 = event-data() -> ()  [unwired: 1 in, 2 out]
        }
        event "Create Cross Cal?", "Save Cross Cal?": Value Change {
          # "Average of STFT"
          # "Create cross cal"
          n105 = event-data() -> ()  [unwired: 1 in, 3 out]
          n106 = Index Array(array=w271) -> (element=w272:T13)  [unwired: 1 in]
          n107 = Unbundle By Name(w272) -> ("A/D info.# lines per scan"=w270:u16)
          n108 = for {
            tunnel: w282 -> [w305] mode=indexing
            tunnel: w281 -> [w304] mode=indexing
            tunnel: [w303] -> w284 mode=indexing
            tunnel: [w302] -> w283 mode=indexing
            tunnel: "Avg #" -> [w301]
            n109 = call "AvrLines.vi"("Avg #"=w301, "intercept (b) in"=w305, "midband fit in"=w304) -> ("intercept avr"=w303:dbl[], "midband avr"=w302:dbl[])  [unwired: 1 in, 2 out]
          }
          n110 = Array Size(array=w271) -> (size(s)=w269:i32)
          n111 = Index Array(array=w260, index=1) -> (element=w266:dbl)
          n112 = Index Array(array=w260) -> (element=w265:dbl)  [unwired: 1 in]
          n113 = Multiply(x=w269, y=w270) -> (x*y=w268:i32)
          n114 = Subtract(x=w266, y=w265) -> (x-y=w264:dbl)
          n115 = Divide(x=w273, y=w268) -> (x/y=w261:dbl[][])
          n116 = expression code="10*log(x)"(w261) -> (w259:dbl[][])
          "spe vs depth" <- w259
          n117 = Transpose 2D Array(2D array=w284) -> (transposed array=w287:dbl[][])
          n118 = Transpose 2D Array(2D array=w283) -> (transposed array=w286:dbl[][])
          n119 = for {
            tunnel: w286 -> [w300] mode=indexing
            tunnel: w287 -> [w299] mode=indexing
            tunnel: [w298] -> w285 mode=indexing
            tunnel: [w297] -> w278 mode=indexing
            n120 = call-poly <vilib>:"Mean.vi"("X"=w300) -> ("mean"=w297:dbl)  [unwired: 1 out]
            n121 = call-poly <vilib>:"Mean.vi"("X"=w299) -> ("mean"=w298:dbl)  [unwired: 1 out]
          }
          n122 = Bundle("x-y"=0.0, w264, w259) -> (→"Waveform Graph":cluster{"x-y":dbl, dbl, dbl[][]})  [unwired: 1 in]
          n123 = Build Array(w278, w285) -> (w277:dbl[][])
          "Cross Cal" <- w277
          n124 = for {
            tunnel: w277 -> [w294] mode=indexing
            tunnel: [w292] -> w276 mode=indexing
            tunnel: "AVG pts" -> [w291]
            tunnel: "start avg" -> [w290]
            n125 = Array Subset(array=w294, index=w290, length=w291) -> (w293:dbl[])
            n126 = call-poly <vilib>:"Mean.vi"("X"=w293) -> ("mean"=w292:dbl)  [unwired: 1 out]
          }
          "avg" <- w276
          n127 = Build Array (concatenate)(w260, w259) -> (w258:dbl[][])
          n128 = case shown="True" "Save Cross Cal?" {
            tunnel: w277 -> [_ w295]
            frame False {
            }
            frame True {
              n129 = call-poly <vilib>:"Write Delimited Spreadsheet.vi"("2D data"=w295, "transpose? (no:F)"=TRUE) -> ()  [unwired: 12 in, 2 out]
            }
          }
          n130 = case shown="True" "Save STFT AVG" {
            tunnel: w258 -> [_ w289]
            frame False {
            }
            frame True {
              n131 = call-poly <vilib>:"Write Delimited Spreadsheet.vi"("2D data"=w289, "transpose? (no:F)"=TRUE) -> ()  [unwired: 12 in, 2 out]
            }
          }
        }
        event "Save Raw Results?": Value Change {
          n132 = event-data() -> ()  [unwired: 1 in, 5 out]
          n133 = local read "Range Params"() -> (w307:T9)
          n134 = for {
            tunnel: w314 -> [w323] mode=indexing
            tunnel: "Raw Data Formats" -> [w322]
            tunnel: w307 -> [w321]
            tunnel: w312 -> [w320] mode=indexing
            tunnel: w311 -> [w315] mode=indexing
            tunnel: "Final Sector Image Size" -> [w319]
            tunnel: w310 -> [w318] mode=indexing
            tunnel: w309 -> [w317] mode=indexing
            tunnel: w308 -> [w316] mode=indexing
            n135 = call "SaveParamImages.vi"("Directory Parh"=w320, "Data Formats"=w322, "file name"=w323, "Range Params"=w321, "slope"=w318, "Header In"=w315, "intercept"=w317, "midband fit"=w316, "Final Image Size"=w319) -> ()  [unwired: 2 in, 5 out]
          }
        }
        event "CQPrams": Value Change {
          n136 = event-data() -> ()  [unwired: 1 in, 5 out]
          n137 = Bundle By Name(cluster="CQPrams", "Data System params.sample freq (MHz)"=w326, "Data System params.pts in window"=w325) -> (w324:T8)
          n138 = for {
            tunnel: w324 -> [w340]
            tunnel: w328 -> [w339] mode=indexing
            tunnel: w332 -> [w338] mode=indexing
            tunnel: w331 -> [w337] mode=indexing
            tunnel: w330 -> [w336] mode=indexing
            tunnel: w329 -> [w335] mode=indexing
            n139 = call "CQ2Image.vi"("CQPrams"=w340, "name"=w339, "Tranducer Info"=w335, "midband fit"=w336, "slope"=w337, "appended path"=w338) -> ("radius (micron)"=→"radius (micron)":sgl[][], "CQ^2"=→"CQ^2":ext[][])  [unwired: 2 out]
          }
        }
        event "Simple BMP": Value Change {
          n140 = event-data() -> ()  [unwired: 1 in, 5 out]
          n141 = for {
            tunnel: w341 -> [w351] mode=indexing
            tunnel: w342 -> [w343] mode=indexing
            w349 = 8
            n142 = invoke on="raw data" class="IntensityGraph (strict)" method="Get Image"("image depth"=w349) -> ("image data"=w346:T23)  [unwired: 5 in, 5 out]
            n143 = invoke on="midband fit" class="IntGraph (strict)" method="Get Image"("image depth"=w349) -> ("image data"=w345:T23)  [unwired: 5 in, 5 out]
            n144 = Concatenate Strings(w351, ".fun.bmp") -> (w347:string)
            n145 = call "Merge BMP.vi"("image two"=w345, "image one"=w346) -> ("Merged"=w344:T23)
            n146 = Build Path(base path=w343, name or relative path=w347) -> (appended path=w350:path)
            n147 = call <vilib>:"Write BMP File.vi"("image data"=w344, "path to BMP file"=w350) -> ()  [unwired: 1 in, 9 out]
          }
        }
        event "Create Score Image?", "thresholds", "Data Set", "PSA Value": Value Change {
          n148 = event-data() -> ()  [unwired: 1 in, 5 out]
          n149 = Index Array(array=w364, index="Data Set") -> (element=w363:string)
          n150 = local read "Final Sector Image Size"() -> (w373:T10)
          n151 = local write "Current File"(w363) -> ()
          n152 = Index Array(array=w367, index (dim 0)="Data Set") -> (element=w353:dbl[][])  [unwired: 2 in]
          n153 = Index Array(array=w366, index (dim 0)="Data Set") -> (element=w354:dbl[][])  [unwired: 2 in]
          n154 = Index Array(array=w365, index="Data Set") -> (element=w352:T13)
          n155 = Index Array(array=w358, index (dim 0)="Data Set") -> (element=w357:dbl[][])  [unwired: 2 in]
          n156 = local write "midband fit"(w354) -> ()
          n157 = local write "intercept"(w353) -> ()
          n158 = local write "Sector as data array"(w357) -> ()
          n159 = call "EncodeInLine.vi"("Look Up Table"="Look Up Table", "Final Sector Image Size"=w373, "Bypass Sector?"="Bypass Sector?", "Range Params"="Range Params", "Header In"=w352, "PSA Value"="PSA Value", "intercept"=w353, "thresholds"="thresholds", "midband fit"=w354) -> ("Score Sector image"=w362:dbl[][], "Colored MB"=→"Col midband":dbl[][], "Colored Score"=→"Col scores":dbl[][], "Range Params in LUT"=→"Range Params in LUT":T9)  [unwired: 1 in, 6 out]
          "NN Score" <- w362
          n160 = Array Max & Min(array=w362) -> (max value=→"max value":dbl, min value=→"min value":dbl)  [unwired: 2 out]
        }
        event "Save Score Dat?": Value Change {
          n161 = event-data() -> ()  [unwired: 1 in, 5 out]
          n162 = local read "Final Sector Image Size"() -> (w380:T10)
          n163 = local read "Range Params"() -> (w376:T9)
          n164 = local read "Look Up Table"() -> (w377:path)
          n165 = local read "thresholds"() -> (w378:T12)
          n166 = local read "PSA Value"() -> (w379:dbl)
          n167 = for {
            tunnel: w385 -> [w400] mode=indexing
            tunnel: w384 -> [w399] mode=indexing
            tunnel: w376 -> [w398]
            tunnel: w380 -> [w397]
            tunnel: w383 -> [w386] mode=indexing
            tunnel: w382 -> [w396] mode=indexing
            tunnel: w381 -> [w395] mode=indexing
            tunnel: w379 -> [w391]
            tunnel: w378 -> [w390]
            tunnel: w377 -> [w389]
            tunnel: "Color Table" -> [w388]
            n168 = call "EncodeInLine.vi"("Look Up Table"=w389, "Final Sector Image Size"=w397, "Range Params"=w398, "Header In"=w386, "PSA Value"=w391, "intercept"=w396, "thresholds"=w390, "midband fit"=w395) -> ("Scale Score"=w392:dbl[][], "Colored MB"=w394:dbl[][], "colored Int"=w393:dbl[][], "Colored Score"=w387:dbl[][])  [unwired: 2 in, 6 out]
            n169 = call "SaveScoreImages.vi"("Color Table"=w388, "Save Directory"=w400, "FileName"=w399, "Colored Score"=w387, "colored Int"=w393, "Colored MB"=w394, "Scaled Score"=w392) -> ()  [unwired: 5 out]
          }
        }
        event "Rescale Thresh": Value Change {
          n170 = event-data() -> ()  [unwired: 1 in, 5 out]
          n171 = local read "max value"() -> (w402:dbl)
          n172 = local read "min value"() -> (w401:dbl)
          n173 = Round Toward +Infinity(x=w402) -> ()  [unwired: 1 out]
          n174 = Round Toward -Infinity(1:w401) -> ()  [unwired: 1 out]
          n175 = property on="T1" class="Slide (strict)"("Scale.Maximum"=w402, "Scale.Minimum"=w401) -> ()  [unwired: 2 in, 2 out]
          n176 = property on="T2" class="Slide (strict)"("Scale.Maximum"=w402, "Scale.Minimum"=w401) -> ()  [unwired: 2 in, 2 out]
          n177 = property on="T3" class="Slide (strict)"("Scale.Maximum"=w402, "Scale.Minimum"=w401) -> ()  [unwired: 2 in, 2 out]
          n178 = property on="T4" class="Slide (strict)"("Scale.Maximum"=w402, "Scale.Minimum"=w401) -> ()  [unwired: 2 in, 2 out]
          n179 = property on="T5" class="Slide (strict)"("Scale.Maximum"=w402, "Scale.Minimum"=w401) -> ()  [unwired: 2 in, 2 out]
        }
        event "Select directory with EYE files": Value Change {
          n180 = event-data() -> ()  [unwired: 1 in, 6 out]
        }
        event "Calculate TTIs": Value Change {
          n181 = event-data() -> ()  [unwired: 1 in, 6 out]
          n182 = Not Equal To 0?(x=w405) -> (x != 0?=w404:bool)
        }
        event "ExitSendCmd": Value Change {
          w406 = TRUE
          n183 = event-data() -> ()  [unwired: 1 in, 5 out]
        }
        event "Final Sector Image Size": Value Change {
          # "find distance bewteen pixels."
          n184 = event-data() -> ("NewVal"=w410:T10)  [unwired: 1 in, 4 out]
          n185 = Unbundle By Name(w407) -> ("X right"=w415:dbl, "X left"=w413:dbl, "Y high"=w412:dbl, "Y low"=w414:dbl)
          n186 = Unbundle By Name(w410) -> ("x"=w411:i32, "y"=w417:i32)
          n187 = Subtract(x=w415, y=w413) -> (x-y=w418:dbl)
          n188 = Subtract(x=w412, y=w414) -> (x-y=w416:dbl)
          n189 = Divide(x=w416, y=w417) -> (x/y=w408:dbl)
          n190 = Divide(x=w418, y=w411) -> (x/y=w409:dbl)
          n191 = local write "inc x (mm)"(w409) -> ()
          n192 = local write "inc y (mm)"(w408) -> ()
        }
      }
    }
  }
